vi "AI端口_油压2.vi"() -> ()   [LabVIEW 2013]
panel:
  out "油压2":tag="Dev1/ai2"
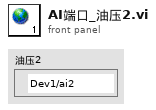
[diagram p1: front panel]
diagram:
